vi "MPM_Get_READ_Power_for_Module.vi"(8 "error in (no error)":errorcluster, 10 "moduleNumber":i32, 11 ".NET Reference in":refnum<k24>) -> (0 "error out":errorcluster, 1 "powers out":dbl[](array[numeric]), 3 "Reference out":refnum<k24>)   [LabVIEW 2017]
uses:
  LV_IL_Sample/DLL/InstrumentDLL.dll
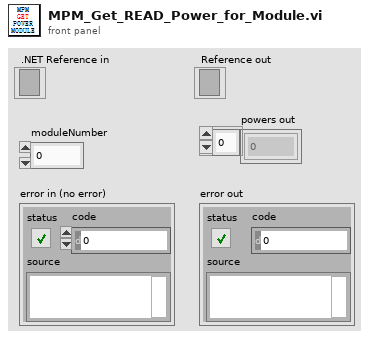
[diagram p1: front panel]
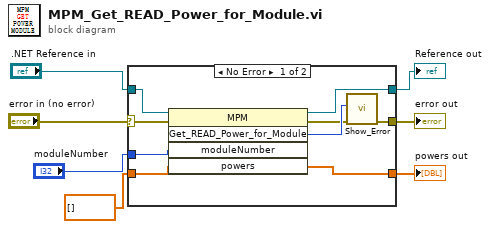
[diagram p0: block diagram]
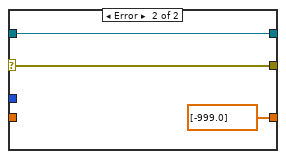
[diagram p2: hidden frame]
diagram:
  n1 = case shown="No Error" "error in (no error)" {
    selector: "error in (no error)" -> [w8 w18]
    tunnel: [w16 dbl[] [-999.0] ("powers")] -> w7
    tunnel: "moduleNumber" -> [w15 _]
    tunnel: ".NET Reference in" -> [w14 w19]
    tunnel: [w13 w19] -> w4
    tunnel: dbl[] [] ("powers") -> [w12 _]
    tunnel: [w9 w18] -> w2
    frame No Error {
      n2 = invoke on="调用节点" class="MPM" method="Get_READ_Power_for_Module"(reference=w14, error in=w8, "moduleNumber"=w15, "powers"=w12) -> (reference out=w13:refnum<k24>, error out=w10:errorcluster, "Get_READ_Power_for_Module"=w11:i32, "powers"=w16:dbl[])  [unwired: 1 in, 1 out]
      n3 = call "Show_Error.vi"("error in (no error)"=w10, "Error"=w11) -> ("error out"=w9:errorcluster)  [unwired: 9 in]
    }
    frame Error {
    }
  }
  "powers out" <- w7
  "Reference out" <- w4
  "error out" <- w2
